vi "pid_main.vi"(5 "limits":T5={"upperLimit"=2.0, "lowerLimit"=0.0}, 6 "ready for output (T)":bool=TRUE, 7 "manualMotion":T1, 8 "input valid":bool=TRUE, 9 "liftOffParams":T3={"liftHeight"=0.0498046875, "disengagePos"=-1.0, "liftOff"=FALSE} {"disengagePos" format="%#_28g"}, 10 "fbParams":T4={"enable"=FALSE, "setPoint"=0.001007080078125, "pGain"=0.0, "iGain"=0.10000038146972656, "gainScale"=0}, 11 "input":fxp<+/-,24,16>) -> (0 "output valid":bool, 3 "output":T2, 4 "ready for input":bool)   [LabVIEW 2016]
uses:
  <vilib>/rvi/FXPMathLib/FxpAdd/XNode/nifxpmath_Add.xnode
  <vilib>/rvi/FXPMathLib/FxpInterpret/XNode/nifxpmath_Interpret.xnode
  <vilib>/rvi/FXPMathLib/FxpSub/XNode/nifxpmath_Sub.xnode
  <vilib>/rvi/FXPMathLib/FxpMul/XNode/nifxpmath_Multiplier.xnode
  <vilib>/rvi/FXPMathLib/sim/FxpSim.dll
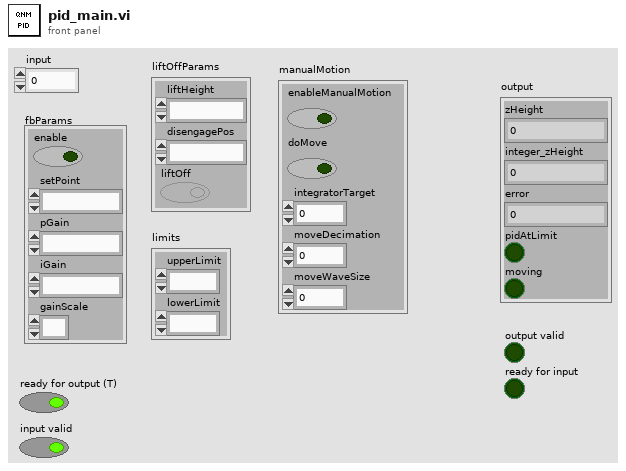
[diagram p1: front panel]
types:
  T1 = cluster{"enableManualMotion":bool, "doMove":bool, "integratorTarget":fxp<+/-,22,2>, "moveDecimation":u16, "moveWaveSize":u16}
  T2 = cluster{"zHeight":fxp<+/-,28,1>, "integer_zHeight":i16, "error":fxp<+/-,25,2>, "pidAtLimit":bool, "moving":bool}
  T3 = cluster{"liftHeight":fxp<+/-,15,4>, "disengagePos":fxp<+/-,22,1>, "liftOff":bool}
  T4 = cluster{"enable":bool, "setPoint":fxp<+/-,17,1>, "pGain":fxp<+/-,20,4>, "iGain":fxp<+/-,20,1>, "gainScale":i8}
  T5 = cluster{"upperLimit":fxp<+/-,28,4>, "lowerLimit":fxp<+/-,28,4>}
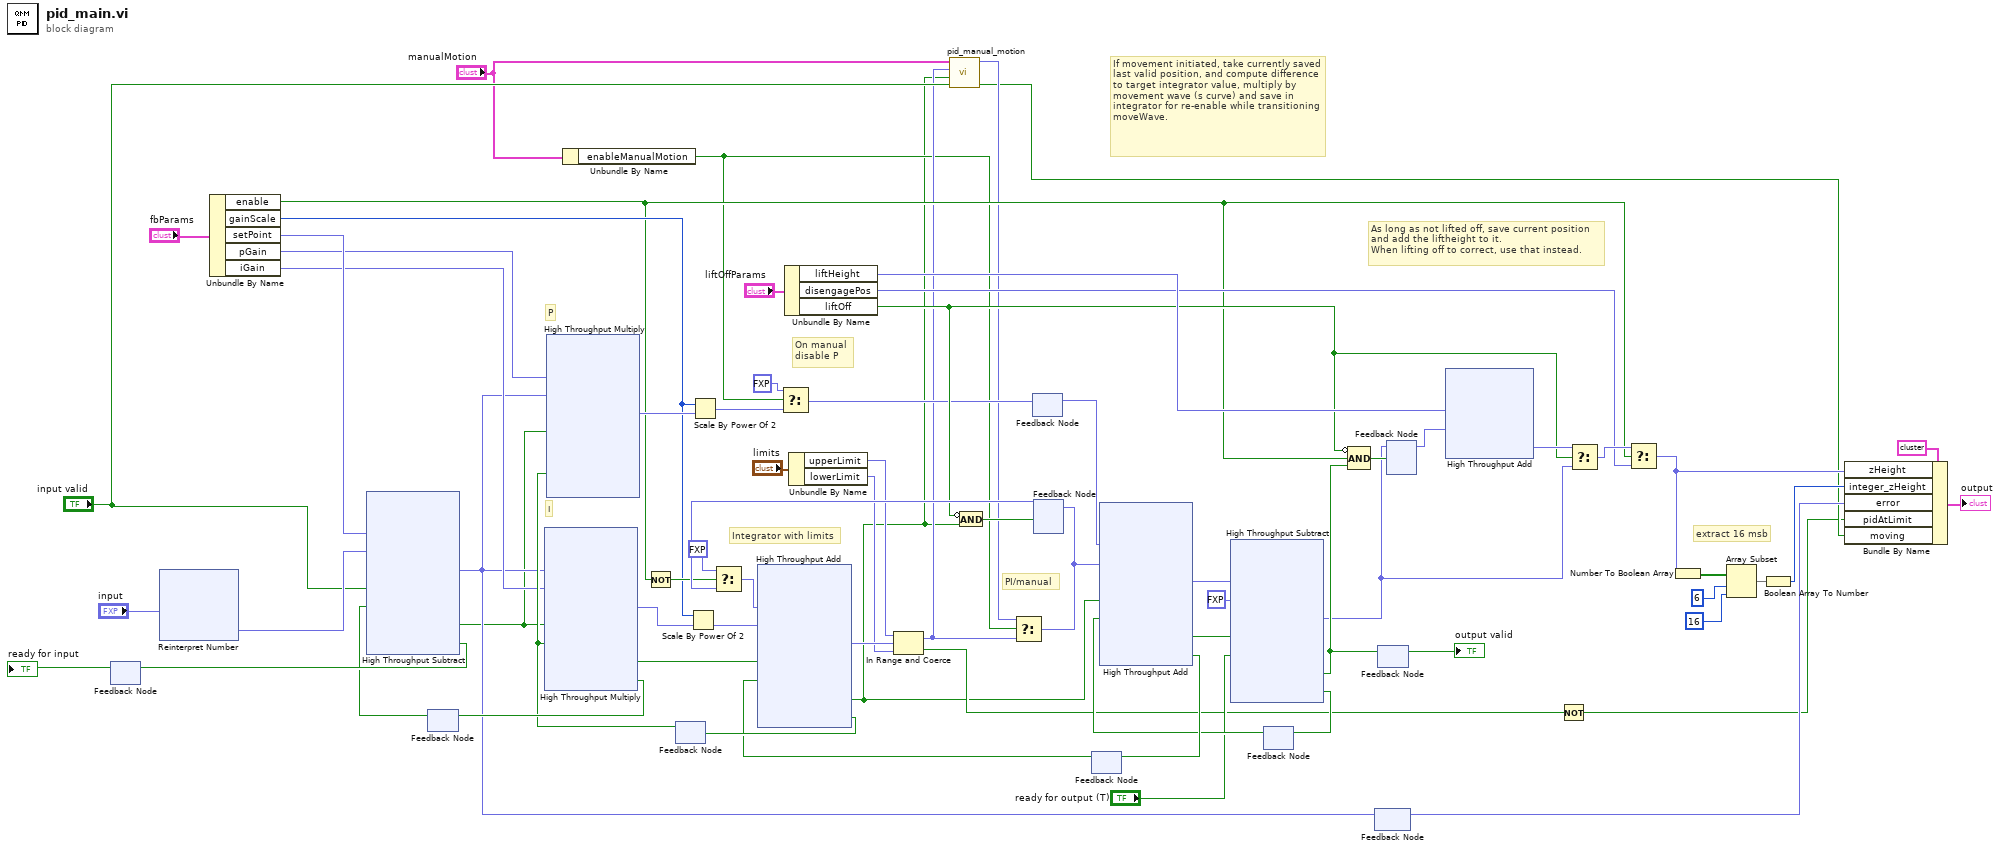
[diagram p0: block diagram]
diagram:
  # "On manual\ndisable P"
  # "PI/manual"
  # "I"
  # "P"
  # "If movement initiated, take currently saved last valid position, and compute difference to target integrator value, multiply by movement wave (s curve) and save in integrator for re-enable while transitioning moveWave."
  # "Integrator with limits"
  # "As long as not lifted off, save current position\nand add the liftheight to it.\nWhen lifting off to correct, use that instead."
  # "extract 16 msb"
  n1 = feedback #1() -> (→"ready for input":bool)  [unwired: 1 in]
  n2 = xnode "Reinterpret Number"("x"="input") -> ("y"=w39:fxp<+/-,24,1>)
  n3 = Unbundle By Name("fbParams") -> ("enable"=w20:bool, "gainScale"=w30:i8, "setPoint"=w33:fxp<+/-,17,1>, "pGain"=w32:fxp<+/-,20,4>, "iGain"=w31:fxp<+/-,20,1>)
  n4 = feedback #2() -> (w68:bool)  [unwired: 1 in]
  n5 = xnode ("High Throughput Subtract")("x"=w33, "y"=w39, "input valid"="input valid", "ready for output (T)"=w68) -> ("x-y"=w22:fxp<+/-,25,2>, "output valid"=w1:bool, "ready for input"=w71:bool)
  n6 = feedback-in #1(w71) -> ()
  n7 = Unbundle By Name("manualMotion") -> ("enableManualMotion"=w5:bool)
  n8 = Not(x=w20) -> (.not. x?=w40:bool)
  n9 = feedback #3() -> (w62:bool)  [unwired: 1 in]
  n10 = xnode ("High Throughput Multiply")("x"=w22, "y"=w31, "input valid"=w1, "ready for output (T)"=w62) -> ("x*y"=w66:fxp<+/-,32,2>, "output valid"=w61:bool, "ready for input"=w69:bool)
  n11 = feedback-in #2(w69) -> ()
  n12 = xnode ("High Throughput Multiply")("x"=w32, "y"=w22, "input valid"=w1, "ready for output (T)"=w62) -> ("x*y"=w57:fxp<+/-,32,2>)  [unwired: 2 out]
  n13 = Scale By Power Of 2(n=w30, x=w66) -> (x*2^n=w36:fxp<+/-,32,2>)
  n14 = Scale By Power Of 2(n=w30, x=w57) -> (x*2^n=w35:fxp<+/-,32,2>)
  n15 = Select(t=fxp<+/-,32,2> 0.0, s=w5, f=w35) -> (s? t:f=w13:fxp<+/-,32,2>)
  n16 = Unbundle By Name("liftOffParams") -> ("liftHeight"=w26:fxp<+/-,15,4>, "disengagePos"=w25:fxp<+/-,22,1>, "liftOff"=w24:bool)
  n17 = Unbundle By Name("limits") -> ("upperLimit"=w58:fxp<+/-,28,4>, "lowerLimit"=w59:fxp<+/-,28,4>)
  n18 = feedback #4() -> (w50:fxp<+/-,32,2>)  [unwired: 1 in]
  n19 = feedback-in #4(w13) -> ()
  n20 = feedback #5() -> (w64:fxp<+/-,32,4>)  [unwired: 1 in]
  n21 = Select(t=fxp<+/-,32,4> 0.0 ("x+y"), s=w40, f=w64) -> (s? t:f=w65:fxp<+/-,32,4>)
  n22 = feedback #6() -> (w14:bool)  [unwired: 1 in]
  n23 = xnode ("High Throughput Add")("x"=w65, "y"=w36, "input valid"=w61, "ready for output (T)"=w14) -> ("x+y"=w67:fxp<+/-,32,4>, "output valid"=w4:bool, "ready for input"=w63:bool)
  n24 = feedback-in #3(w63) -> ()
  n25 = In Range and Coerce(upper limit=w58, x=w67, lower limit=w59) -> (coerced(x)=w8:fxp<+/-,32,4>, In Range?=w17:bool)
  n26 = call "pid_manual_motion.vi"("inputValid"="input valid", "lastPosValid"=w4, "lastPos"=w8, "manualMotion"="manualMotion") -> ("moving"=w3:bool, "output"=w9:fxp<+/-,32,4>)  [unwired: 5 in, 1 out]
  n27 = Compound Arithmetic op=AND(invert w24, w4) -> (w10:bool)
  n28 = Select(t=w9, s=w5, f=w8) -> (s? t:f=w6:fxp<+/-,32,4>)
  n29 = feedback-in #5(w6, w10) -> ()
  n30 = feedback #7() -> (w51:bool)  [unwired: 1 in]
  n31 = xnode ("High Throughput Add")("x"=w50, "y"=w6, "input valid"=w4, "ready for output (T)"=w51) -> ("x+y"=w54:fxp<+/-,26,3>, "output valid"=w53:bool, "ready for input"=w56:bool)
  n32 = feedback-in #6(w56) -> ()
  n33 = xnode ("High Throughput Subtract")("x"=w54, "y"=fxp<+,1,1> 1.0, "input valid"=w53, "ready for output (T)"="ready for output (T)") -> ("x-y"=w37:fxp<+/-,22,1>, "output valid"=w41:bool, "ready for input"=w52:bool)
  n34 = feedback-in #7(w52) -> ()
  n35 = Compound Arithmetic op=AND(invert w24, w20, w41) -> (w46:bool)
  n36 = feedback #8() -> (w21:fxp<+/-,25,2>)  [unwired: 1 in]
  n37 = feedback-in #8(w22) -> ()
  n38 = feedback #9() -> (→"output valid":bool)  [unwired: 1 in]
  n39 = feedback-in #9(w41) -> ()
  n40 = feedback #10() -> (w44:fxp<+/-,22,1>)  [unwired: 1 in]
  n41 = feedback-in #10(w37, w46) -> ()
  n42 = xnode ("High Throughput Add")("x"=w26, "y"=w44) -> ("x+y"=w43:fxp<+/-,22,1>)
  n43 = Not(x=w17) -> (.not. x?=w2:bool)
  n44 = Select(t=w43, s=w24, f=w37) -> (s? t:f=w42:fxp<+/-,22,1>)
  n45 = Select(t=w42, s=w20, f=w25) -> (s? t:f=w15:fxp<+/-,22,1>)
  n46 = Number To Boolean Array(number=w15) -> (Boolean array=w47:bool[])
  n47 = Array Subset(array=w47, index=6, length=16) -> (w45:bool[])
  n48 = Boolean Array To Number(Boolean array=w45) -> (number=w23:i16)
  n49 = Bundle By Name(cluster=T2 {"zHeight"=0.0, "integer_zHeight"=0, "error"=0.0, "pidAtLimit"=FALSE, "moving"=FALSE} ("output"), "zHeight"=w15, "integer_zHeight"=w23, "error"=w21, "pidAtLimit"=w2, "moving"=w3) -> (→"output":T2)
